vi "AddNetDevice.vi"(0 "Handle In":u64[](array[numeric]), 1 "error in":errorcluster, 5 "Proto":i32(ring) items=["TCP", "UDP", "RTUOverTCP", "RTUOverUDP"], 7 "Address":string="127.0.0.1", 9 "Port":u16=502, 11 "Device ID":u8(ring) items=["4800"=192, "9600"=128, "19200"=0, "38400"=0, "1"=0, "115200"=0]) -> (3 "error out":errorcluster, 4 "Handle Out":u64[](array[numeric]), 6 "Result":i32)   [LabVIEW 2020, in "SnapMB.lvlib"]
uses:
  SnapMB.lvlib
  windows/snapmb.dll
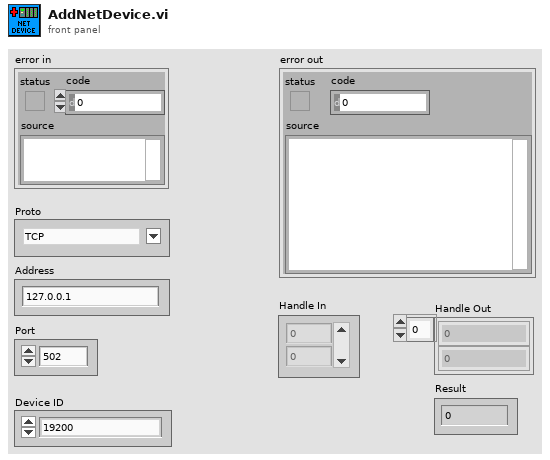
[diagram p1: front panel]
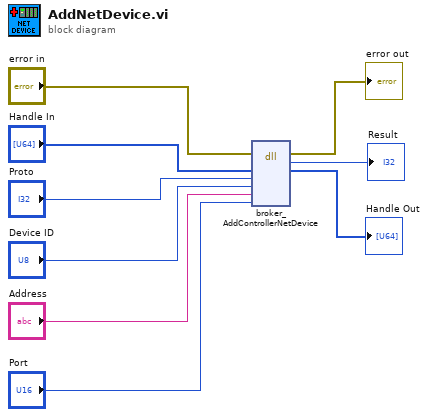
[diagram p0: block diagram]
diagram:
  n1 = dll-call lib="D:/SnapMB/LabView/lib/windows/snapmb.dll" fn="broker_AddControllerNetDevice"(error in="error in", "Broker"="Handle In", "Proto"="Proto", "DeviceID"="Device ID", "Address"="Address", "Port"="Port") -> (error out=→"error out":errorcluster, "return type"=→"Result":i32, "Broker"=→"Handle Out":u64[])  [unwired: 6 in, 1 out]
